vi "Retreive Path From List.vi"(7 "Error if Not Found":T1, 8 "error in (no error)":errorcluster, 10 "Name":string, 11 "List in":variant) -> (0 "error out":errorcluster, 2 "Path":path, 3 "List out":variant)   [LabVIEW 2018, in "Scripting.lvlib"]
uses:
  Scripting.lvlib
  Error-Codes.ctl
  Bundle-Error.vi
  Error-Offset.vi
  <vilib>/Utility/error.llb/Error Cluster From Error Code.vi
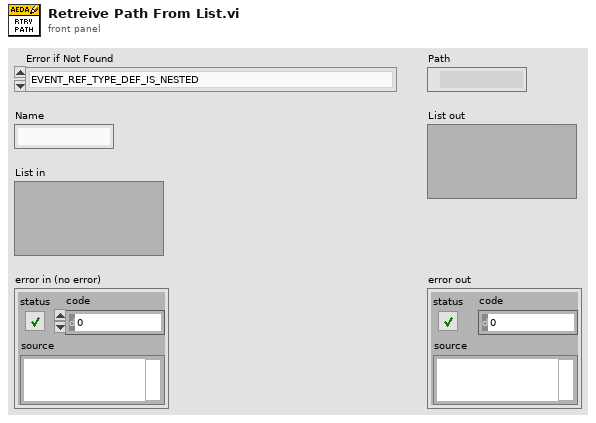
[diagram p1: front panel]
types:
  T1 = typedef "Scripting.lvlib/Error-Codes.ctl" = enum16{"EVENT_REF_TYPE_DEF_IS_NESTED", "EVENT_REF_TYPE_DEF_IS_EMPTY", "EVENT_REF_TYPE_DEF_INCLUDES_NON_REFS", "EVENT_REF_TYPE_INVALID_REPLY_REF", "EVENT_REF_TYPE_REPLY_IS_NOT_TYPE_DEF", "EVENT_REF_TYPE_DEF_IS_NOT_CLUSTER", "EVENT_REF_TYPE_DEF_INVALID_REQ_REPLY_TYPE", "ACTOR_CLASS_PATH_IS_INVALID", "ACTOR_CLASS_LIBRARY_IS_NOT_EDITABLE", "ACTOR_CLASS_CREATE_ENQUEUER_REFS_VI_NOT_FOUND", "MSG_ENQUEUER_REFS_CTL_NOT_FOUND", "ACTOR_CLASS_MAIN_RUN_VI_NOT_FOUND", "ACTOR_CLASS_DESTROY_ENQUEUER_REFS_VI_NOT_FOUND", "CREATE_ENQUEUER_REFS_ERROR_TERMINAL_NOT_FOUND", "CREATE_ENQUEUER_REFS_INVALID_TYPE_DEF", "CREATE_ENQUEUER_REF_NAMEBUNDLER_NOT_FOUND", "CREATE_ENQUEUER_REF_MULTIPLE_NAMEBUNDLERS", "MESSAGES_REF_TYPE_DEF_IS_EMPTY", "MESSAGES_REF_TYPE_DEF_IS_NESTED", "ACTOR_TEMPLATE_CLASS_NOT_FOUND"}
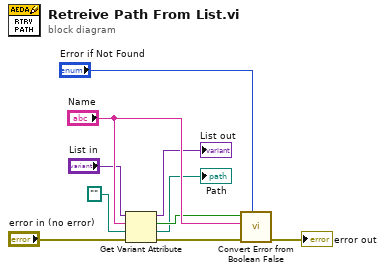
[diagram p0: block diagram]
diagram:
  n1 = Get Variant Attribute(Variant="List in", name="Name", default value (empty Variant)=path "" ("Path"), error in="error in (no error)") -> (duplicate Variant=→"List out":variant, found=w3:bool, value=→"Path":path, error out=w7:errorcluster)
  n2 = call "Convert Error from Boolean False.vi"("Convert to Error Code"="Error if Not Found", "error in (no error)"=w7, "Error Message (\"\")"="Name", "Error Input"=w3) -> ("error out"=→"error out":errorcluster)  [unwired: 7 in]
